vi "TX_多通道FM.vi"() -> ()   [LabVIEW 2019]
uses:
  <vilib>/sound2/lvsound2.llb/Sound File Info (path).vi
  <vilib>/sound2/lvsound2.llb/Sound File Read Open.vi
  <vilib>/Analysis/2dsp.llb/Rational Resample (single channel, DBL).vi
  <vilib>/sound2/lvsound2.llb/Sound File Read (DBL).vi
  <instrlib>/niUSRP/niUSRP Write Tx Data (CDB).vi
  <vilib>/Analysis/NI_AALPro.lvlib
panel:
  in  "Amp.1 2":dbl=1.0 caption="Frequency"
  in  "Freq.1 2":dbl caption="Frequency"
  in  "Amp.1":dbl=1.0 caption="Frequency"
  out "XY Graph 2":cluster{dbl[], dbl[]}(graph)
  in  "Freq.1":dbl=300000.0 caption="Frequency"
  in  "FM deviation(HZ) 2":dbl(slide) scale=0.0..100000.0
  out "Waveform Graph 2":waveform(dbl)(graph)
  in  "path 3":path
  in  "stop":bool
  in  "active antenna":string="TX1"
  out "error out":errorcluster
  out "XY Graph":cluster{dbl[], dbl[]}(graph)
  in  "FM deviation(HZ)":dbl(slide) scale=0.0..100000.0
  out "coerced gain":dbl format="%#_6f"
  out "coerced carrier frequency":dbl=2400000000.0 format="%#_6p"
  out "coerced IQ rate":dbl=200000.0 format="%#_6p"
  in  "gain":dbl format="%#_6f"
  in  "carrier frequency":dbl=2400000000.0 format="%#_6p"
  in  "IQ rate":dbl=200000.0 format="%#_6p"
  in  "IP":refnum<k15>="192.168.10.2"
  in  "number of samples/ch (-1: all)":i32=10000
  out "Waveform Graph":waveform(dbl)(graph)
  in  "path":path
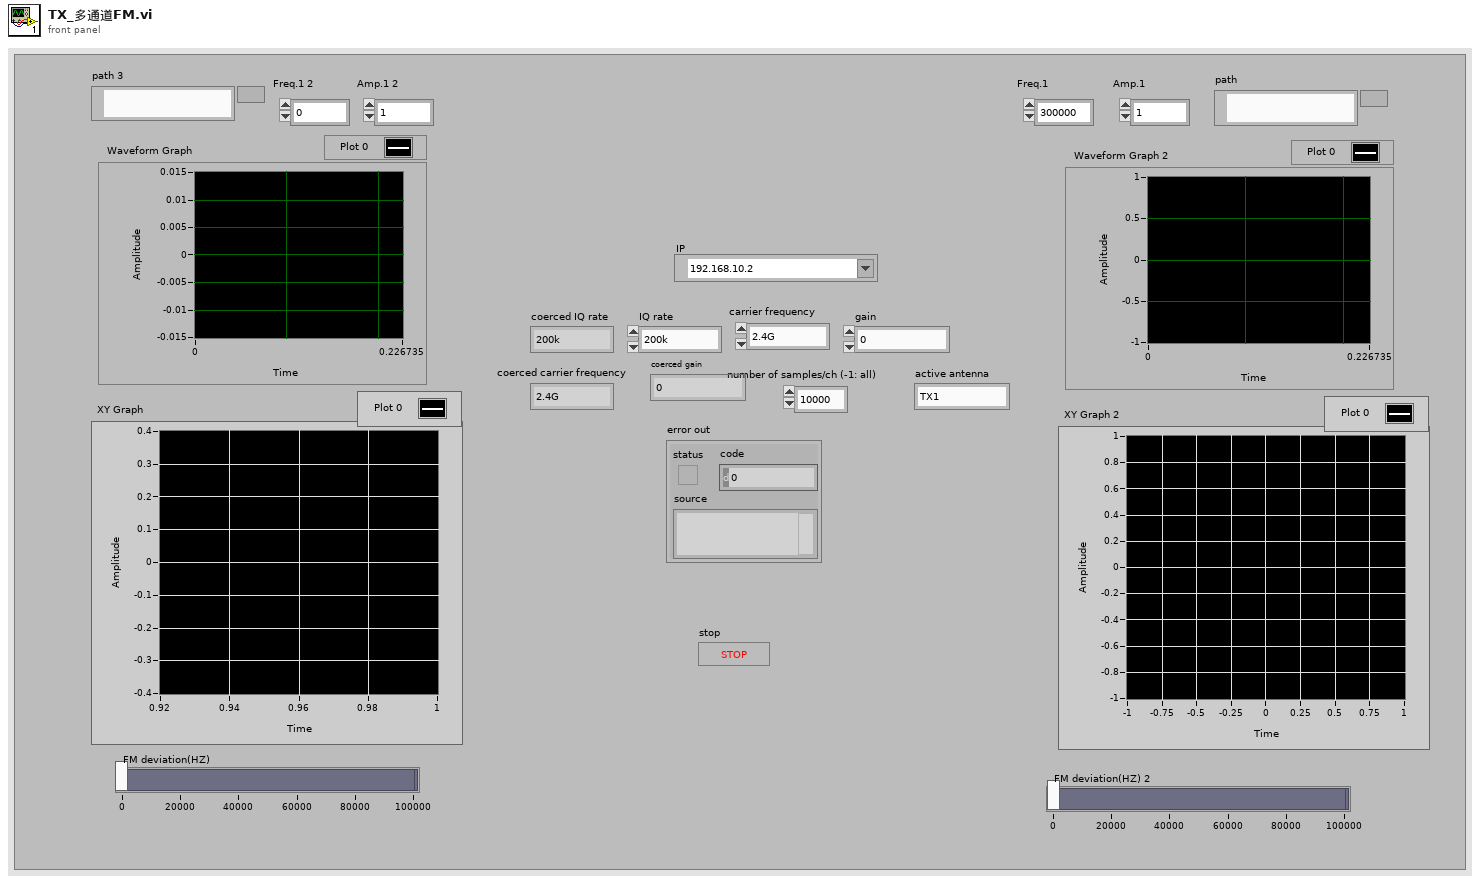
[diagram p1: front panel]
types:
  T1 = typedef "Sound Data Format.ctl" = cluster{"sample rate (S/s)":dbl, "number of channels":i32, "bits per sample":i32}
  T2 = typedef "Sound File Refnum.ctl" = refnum<file>
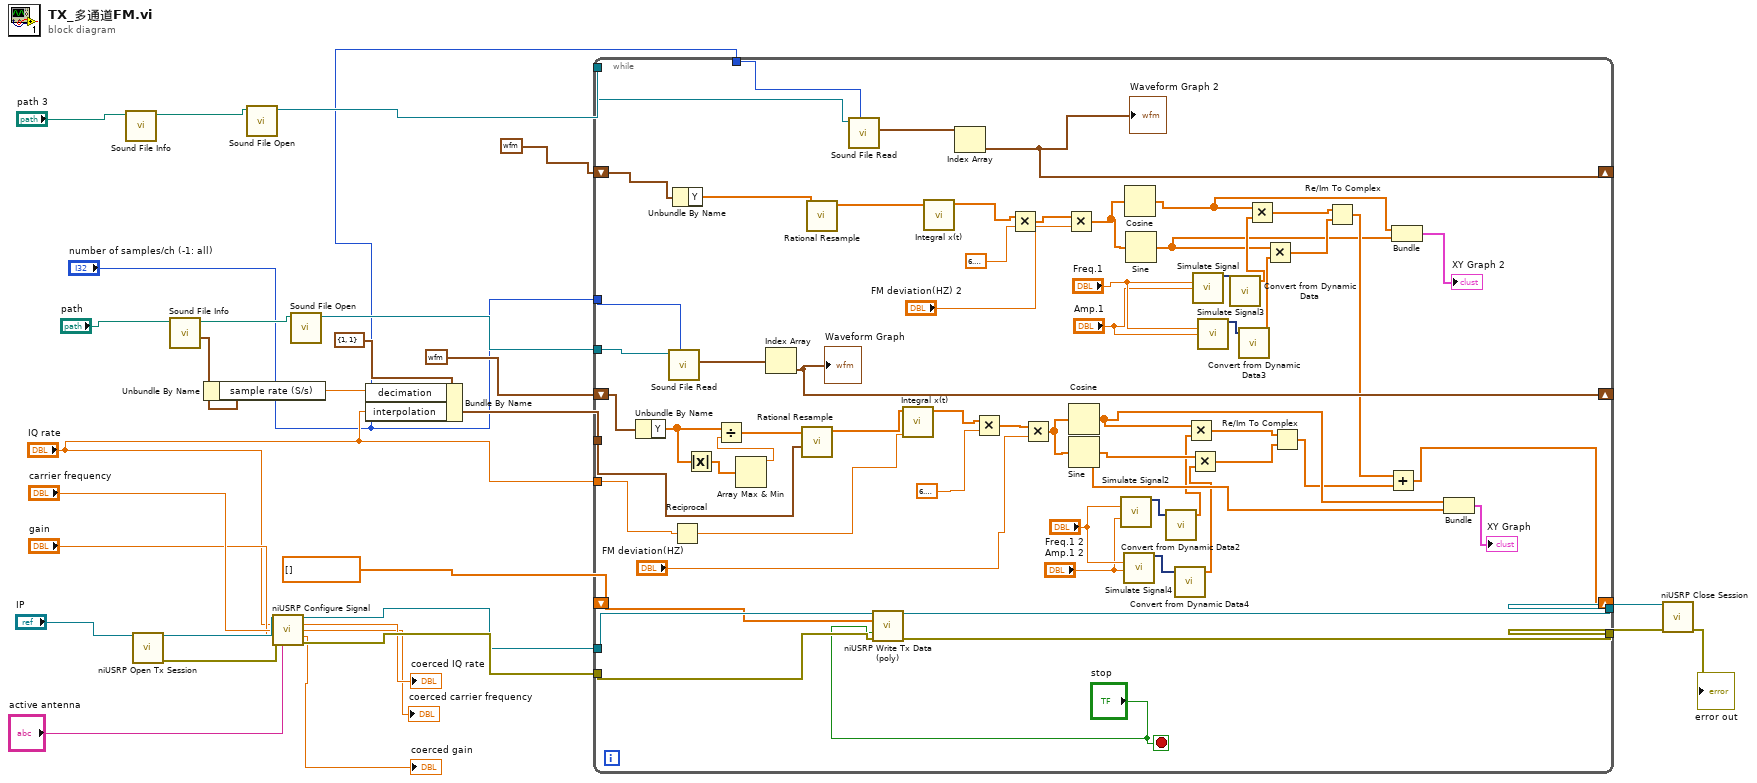
[diagram p0: block diagram]
diagram:
  n1 = call-poly <vilib>:"Sound File Info.vi"("path"="path 3") -> ("path out"=w6:path)  [unwired: 7 in, 3 out]
  n2 = call <instrlib>:"niUSRP Open Tx Session.vi"("device names"="IP") -> ("session handle out"=w25:refnum<k15>, "error out"=w24:errorcluster)  [unwired: 13 in]
  n3 = call-poly <vilib>:"Sound File Info.vi"("path"="path") -> ("sound format"=w12:T1, "path out"=w28:path)  [unwired: 7 in, 2 out]
  n4 = Unbundle By Name(w12) -> ("sample rate (S/s)"=w10:dbl)
  n5 = call-poly <vilib>:"Sound File Open.vi"("path"=w6) -> ("sound file refnum"=w5:T2)  [unwired: 9 in, 1 out]
  n6 = call <instrlib>:"niUSRP Configure Signal.vi"("session handle"=w25, "IQ rate"="IQ rate", "carrier frequency"="carrier frequency", "gain"="gain", "error in (no error)"=w24, "active antenna"="active antenna") -> ("session handle out"=w22:refnum<k15>, "coerced IQ rate"=→"coerced IQ rate":dbl, "coerced carrier frequency"=→"coerced carrier frequency":dbl, "coerced gain"=→"coerced gain":dbl, "error out"=w23:errorcluster)  [unwired: 5 in]
  n7 = call-poly <vilib>:"Sound File Open.vi"("path"=w28) -> ("sound file refnum"=w27:T2)  [unwired: 9 in, 1 out]
  n8 = Bundle By Name(cluster=cluster{"interpolation":i32, "decimation":i32} {"interpolation"=1, "decimation"=1} ("input cluster"), "decimation"=w10, "interpolation"="IQ rate") -> (w11:cluster{"interpolation":i32, "decimation":i32})
  n9 = while {
    tunnel: w27 -> [w90]
    shift-right: [w60] -> _
    shift-left: waveform(dbl) {"t0"=timestamp(0 s since 1904-01-01), "dt"=1.0, "Y"=[]} ("data") -> [w82]
    tunnel: "number of samples/ch (-1: all)" -> [w88]
    tunnel: w23 -> [w87]
    tunnel: w22 -> [w86]
    tunnel: "IQ rate" -> [w85]
    tunnel: [w84] -> w16
    tunnel: [w83] -> w15
    shift-right: [w57] -> _
    shift-left: cdb[] [] ("Array") -> [w74]
    tunnel: w11 -> [w73]
    tunnel: w5 -> [w70]
    tunnel: "number of samples/ch (-1: all)" -> [w69]
    shift-right: [w59] -> _
    shift-left: waveform(dbl) {"t0"=timestamp(0 s since 1904-01-01), "dt"=1.0, "Y"=[]} ("data") -> [w58]
    stop <- "stop" stop-if-true
    n10 = Unbundle By Name(w82) -> ("Y"=w32:dbl[])
    n11 = call-poly <vilib>:"Sound File Read.vi"("number of samples/ch (-1: all)"=w88, "sound file refnum"=w90) -> ("data"=w89:waveform(dbl)[])  [unwired: 5 in, 4 out]
    n12 = Reciprocal(x=w85) -> (1/x=w80:dbl)
    n13 = Unbundle By Name(w58) -> ("Y"=w67:dbl[])
    n14 = Absolute Value(x=w32) -> (abs(x)=w33:dbl[])
    n15 = Array Max & Min(array=w33) -> (max value=w31:dbl)  [unwired: 3 out]
    n16 = Divide(x=w32, y=w31) -> (x/y=w30:dbl[])
    n17 = Index Array(array=w89) -> (element=w60:waveform(dbl))  [unwired: 1 in]
    "Waveform Graph" <- w60
    n18 = call-poly <vilib>:"Rational Resample.vi"("resample factor"=w73, "X"=w30) -> ("Y"=w81:dbl[])  [unwired: 7 in, 2 out]
    n19 = call-poly <vilib>:"Rational Resample.vi"("X"=w67) -> ("Y"=w66:dbl[])  [unwired: 8 in, 2 out]
    n20 = call-poly <vilib>:"Sound File Read.vi"("number of samples/ch (-1: all)"=w69, "sound file refnum"=w70) -> ("data"=w68:waveform(dbl)[])  [unwired: 5 in, 4 out]
    n21 = call-poly <instrlib>:"niUSRP Write Tx Data (poly).vi"("session handle"=w86, "data"=w74, "end of data?"="stop", "error in (no error)"=w87) -> ("session handle out"=w84:refnum<k15>, "error out"=w83:errorcluster)  [unwired: 10 in]
    n22 = call <vilib>:"Integral x(t).vi"("dt"=w80, "X"=w81) -> ("Integral X"=w79:dbl[])  [unwired: 8 in, 1 out]
    n23 = call <vilib>:"Integral x(t).vi"("X"=w66) -> ("Integral X"=w65:dbl[])  [unwired: 9 in, 1 out]
    n24 = Index Array(array=w68) -> (element=w59:waveform(dbl))  [unwired: 1 in]
    "Waveform Graph 2" <- w59
    n25 = Multiply(x=w79, y=6.283185307179586) -> (x*y=w77:dbl[])
    n26 = Multiply(x=w65, y=6.283185307179586) -> (x*y=w62:dbl[])
    n27 = Multiply(x=w77, y="FM deviation(HZ)") -> (x*y=w75:dbl[])
    n28 = Multiply(x=w62, y="FM deviation(HZ) 2") -> (x*y=w61:dbl[])
    n29 = Cosine(x=w75) -> (cos(x)=w41:dbl[])
    n30 = Sine(x=w75) -> (sin(x)=w40:dbl[])
    n31 = call "Simulate Signal2"("Frequency"="Freq.1 2", "Phase"="Amp.1 2") -> ("Sine"=w54:dynamicdata)  [unwired: 12 in, 1 out]
    n32 = call "Simulate Signal4"("Frequency"="Freq.1 2", "Amplitude"="Amp.1 2") -> ("Sine"=w38:dynamicdata)  [unwired: 12 in, 1 out]
    n33 = Cosine(x=w61) -> (cos(x)=w45:dbl[])
    n34 = Sine(x=w61) -> (sin(x)=w44:dbl[])
    n35 = call "Convert from Dynamic Data2"("Dynamic Data Type"=w54) -> ("Array"=w39:dbl[])  [unwired: 3 in]
    n36 = call "Convert from Dynamic Data4"("Dynamic Data Type"=w38) -> ("Array"=w37:dbl[])  [unwired: 3 in]
    n37 = Multiply(x=w41, y=w39) -> (x*y=w43:dbl[])
    n38 = Multiply(x=w40, y=w37) -> (x*y=w42:dbl[])
    n39 = call "Simulate Signal"("Frequency"="Freq.1", "Amplitude"="Amp.1") -> ("Sine"=w56:dynamicdata)  [unwired: 12 in, 1 out]
    n40 = call "Simulate Signal3"("Frequency"="Freq.1", "Amplitude"="Amp.1") -> ("Sine"=w51:dynamicdata)  [unwired: 12 in, 1 out]
    n41 = call "Convert from Dynamic Data"("Dynamic Data Type"=w56) -> ("Array"=w50:dbl[])  [unwired: 3 in]
    n42 = call "Convert from Dynamic Data3"("Dynamic Data Type"=w51) -> ("Array"=w49:dbl[])  [unwired: 3 in]
    n43 = Multiply(x=w45, y=w50) -> (x*y=w48:dbl[])
    n44 = Multiply(x=w44, y=w49) -> (x*y=w47:dbl[])
    n45 = Re/Im To Complex(1:w42, 2:w43) -> (0:w34:cdb[])
    n46 = Re/Im To Complex(1:w47, 2:w48) -> (0:w46:cdb[])
    n47 = Add(x=w46, y=w34) -> (x+y=w57:cdb[])
    n48 = Bundle(w45, w44) -> (→"XY Graph 2":cluster{dbl[], dbl[]})  [unwired: 1 in]
    n49 = Bundle(w41, w40) -> (→"XY Graph":cluster{dbl[], dbl[]})  [unwired: 1 in]
  }
  n50 = call <instrlib>:"niUSRP Close Session.vi"("session handle"=w16, "error in (no error)"=w15) -> ("error out"=→"error out":errorcluster)  [unwired: 13 in]
